vi "Calculate_MecanumDrive.vi"(6 "Rotation":dbl, 7 "Gyro Angle":dbl, 9 "Y":dbl, 10 "X":dbl) -> (0 "Rear Right":dbl, 1 "Rear Left":dbl, 2 "Front Right":dbl, 3 "FrontLeft":dbl)   [LabVIEW 2012]
doc: "Configures the motors for holonomic driving. Holonomic driving allows you to move the robot in any direction without first rotating or maneuvering the robot.\n\nThis VI requires the robot to have either four omni-directional wheels and four motors mounted at 45 degree angles in the four corners of a square frame or to have four mecanum wheels driven by four motors.\n\nThe control input is intended to be connected directly to the X, Y, and Z axes of a joystick. The Y axis is inverted for you.\n\nThis software is licensed. Open the labview\\readme\\WPI Robotics Library Open Source License.txt file for more information."
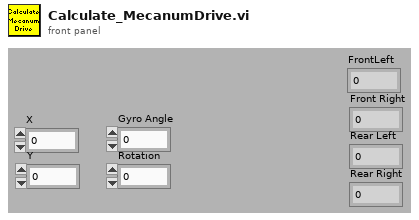
[diagram p1: front panel]
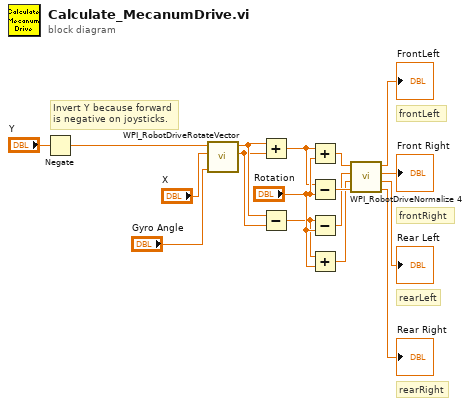
[diagram p0: block diagram]
diagram:
  # "Invert Y because forward is negative on joysticks."
  # "rearLeft"
  # "frontRight"
  # "rearRight"
  # "frontLeft"
  n1 = Negate(x="Y") -> (-x=w1:dbl)
  n2 = call <vilib>:"WPI_RobotDriveRotateVector.vi"("Angle"="Gyro Angle", "X"="X", "Y"=w1) -> ("X'"=w12:dbl, "Y'"=w13:dbl)  [unwired: 7 out]
  n3 = Add(x=w13, y=w12) -> (x+y=w10:dbl)
  n4 = Subtract(x=w13, y=w12) -> (x-y=w8:dbl)
  n5 = Add(x=w10, y="Rotation") -> (x+y=w6:dbl)
  n6 = Subtract(x=w10, y="Rotation") -> (x-y=w11:dbl)
  n7 = Subtract(x=w8, y="Rotation") -> (x-y=w7:dbl)
  n8 = Add(x=w8, y="Rotation") -> (x+y=w9:dbl)
  n9 = call <vilib>:"WPI_RobotDriveNormalize 4.vi"("D"=w11, "C"=w9, "B"=w7, "A"=w6) -> ("D'"=→"Rear Right":dbl, "C'"=→"Rear Left":dbl, "B'"=→"Front Right":dbl, "A'"=→"FrontLeft":dbl)
